vi "StrQueue-Insert (1D).vi"(2 "queue in":string[](array[string]), 4 "string":string[](array[string])) -> (5 "queue out":string[](array[string]))   [LabVIEW 2015]
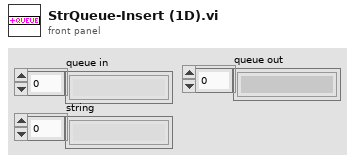
[diagram p1: front panel]
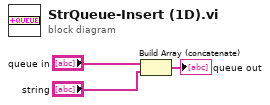
[diagram p0: block diagram]
diagram:
  n1 = Build Array (concatenate)("queue in", "string") -> (→"queue out":string[])
